vi "Test_Install_all_availablePXI.vi"(4 "error in":errorcluster, 7 "Parameter Array in":string[](array[string])) -> (0 "error out":errorcluster, 1 "Result Paragraphs":string[](array[string]), 2 "Pass":bool, 3 "Parameter Array Out":string[](array[string]))   [LabVIEW 2020]
uses:
  <vilib>/nisyscfg/Software 1.2.ctl
  <vilib>/nisyscfg/Component Type.ctl
  <vilib>/nisyscfg/Broken Dependency 1.2.ctl
  <vilib>/nisyscfg/Network Settings Format.ctl
  CommonSubVIs/Framework/Flattened_Array/Test Parameter Enum.ctl
  CommonSubVIs/Framework/Flattened_Array/Get Parameter Value by Name (String).vi
  <vilib>/nisyscfg/Get Filtered Base System Images.vi
  <vilib>/nisyscfg/Format With Base System Image.vi
  <vilib>/nisyscfg/Close (System).vi
  <vilib>/nisyscfg/nisyscfg.lvlib
  <resource>/objmgr/nisysapi.rc
panel:
  in  "Tab Control":enum32{"Connector Pane controls", "The rest"}(tab)
  in  "Network Address":string="10.0.62.162"
  out "Installed Software":T1[](array[typedef]) {"component type" items=["standard", "hidden", "system", "unknown", "startup", "image", "essential"]}
  out "Broken Dependencies":T3[](array[typedef]) {"dependee"."component type" items=["standard", "hidden", "system", "unknown", "startup", "image", "essential"]; "depender"."component type" items=["standard", "hidden", "system", "unknown", "startup", "image", "essential"]}
  in  "Network Settings (reset all adapters)":T4=1 items=["reset all network adapters", "preserve primary, reset others", "preserve all network adapters"]
  out "Base System Image":T1 caption="software" {"component type" items=["standard", "hidden", "system", "unknown", "startup", "image", "essential"]}
  # "This VI is used to install software to the Linux target USEING IPK"
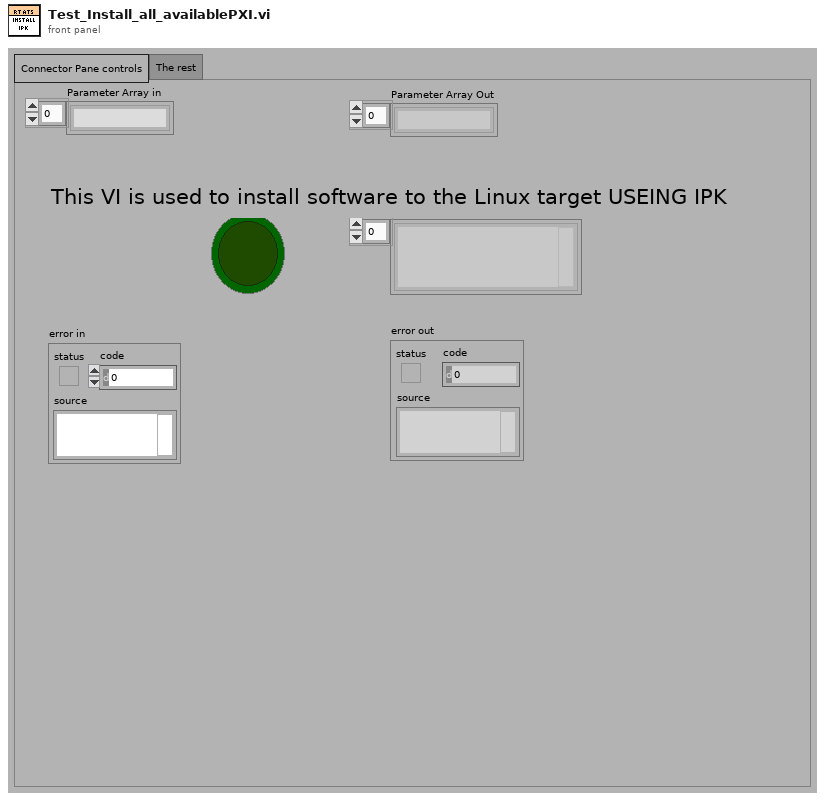
[diagram p1: front panel]
types:
  T1 = typedef "nisyscfg.lvlib/Software 1.2.ctl" = cluster{"title":string, "description":string, "ID":string, "version":string, "component type":T2}
  T2 = typedef "nisyscfg.lvlib/Component Type.ctl" = u32
  T3 = typedef "nisyscfg.lvlib/Broken Dependency 1.2.ctl" = cluster{"depender":T1, "dependee":T1}
  T4 = typedef "nisyscfg.lvlib/Network Settings Format.ctl" = u32
  T5 = typedef "Test Parameter Enum.ctl" = enum16{"Main Test Target IP", "Main Test Target Name", "Main Test Target Alias", "Main Host IP", "Default Target Alias", "Default Target Host Name", "Dafault Target IP Address", "Dafault Target LV Date", "Available Targets", "Target Alias by Index", "Target IP by Alias", "Target IP by  Index", "Current Iteration", "Total Iterations", "Test Project Name", "Current Test Result", "Current Test Name", "Current Test Logical Path", "Test Folder", "Configuration Name", "Configuration Index", "Total Configurations", "Performance Values", "Result Paragraphs", "Connector Pane", "Avoid?", "Avoid Reason", "Case Name", "Case #", "Total Cases", "Case Data", "Disable reason"}
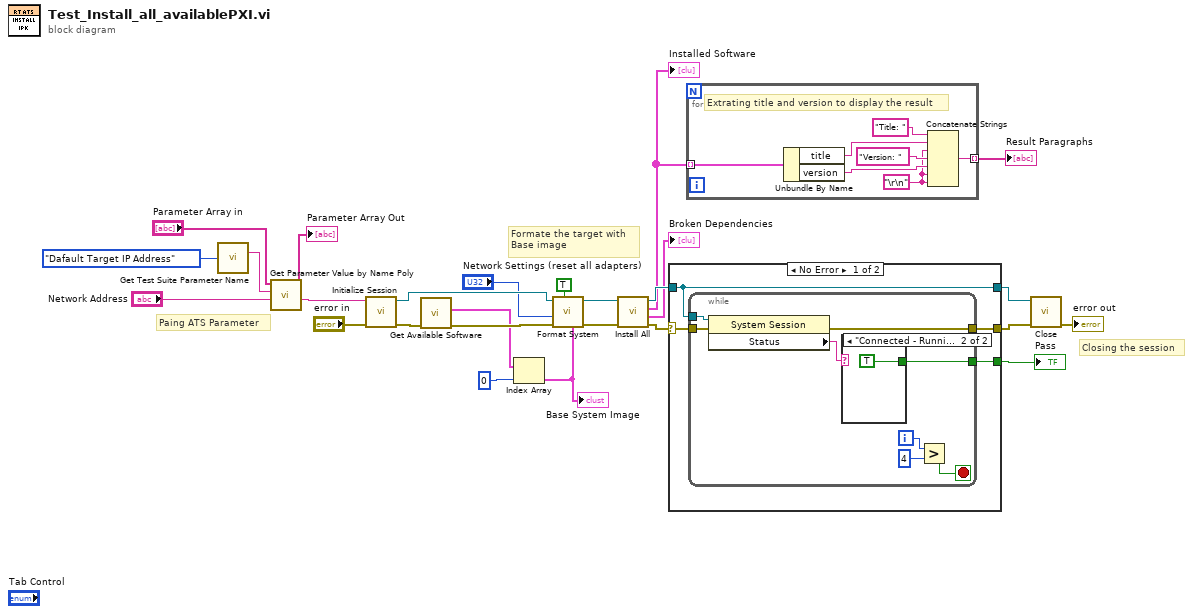
[diagram p0: block diagram]
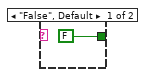
[diagram p2: hidden frame]
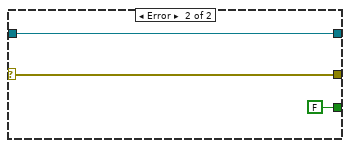
[diagram p3: hidden frame]
diagram:
  # "Closing the session"
  # "Paing ATS Parameter"
  # "Formate the target with \nBase image"
  n1 = call "Get Test Suite Parameter Name.vi"("Test Suite Parameter"=Test_Parameter_Enum."Dafault Target IP Address") -> ("Parameter Name"=w21:string)  [unwired: 13 in, 1 out]
  n2 = call-poly "Get Parameter Value by Name Poly.vi"("Default Value"="Network Address", "Parameter"=w21, "Parameter Array in"="Parameter Array in") -> ("Value"=w11:string, "Parameter Array Out"=→"Parameter Array Out":string[])  [unwired: 5 in, 1 out]
  n3 = call <vilib>:"Initialize Session.vi"("error in (no error)"="error in", "Target (localhost)"=w11) -> ("error out"=w5:errorcluster, "Session out"=w18:refnum<k21>)  [unwired: 8 in]
  n4 = call-poly <vilib>:"Get Available Software.vi"("error in (no error)"=w5) -> ("error out"=w4:errorcluster, "Base System Images"=w3:T1[])  [unwired: 8 in, 1 out]
  n5 = Index Array(array=w3, index=0) -> (element=w1:T1)
  "Base System Image" <- w1
  n6 = call-poly <vilib>:"Format System.vi"("Base System Image"=w1, "Restart Automatically (T)"=TRUE, "error in (no error)"=w4, "Network Settings (reset all adapters)"="Network Settings (reset all adapters)", "Session in"=w18) -> ("error out"=w16:errorcluster, "Session out"=w15:refnum<k21>)  [unwired: 5 in]
  n7 = call <vilib>:"Install All.vi"("error in (no error)"=w16, "Session in"=w15) -> ("error out"=w24:errorcluster, "Broken Dependencies"=→"Broken Dependencies":T3[], "Installed Software"=w7:T1[], "Session out"=w25:refnum<k21>)  [unwired: 6 in]
  "Installed Software" <- w7
  n8 = case shown="No Error" w24 {
    selector: w24 -> [w29 w41]
    tunnel: w25 -> [w27 w43]
    tunnel: [w30 FALSE] -> w26
    tunnel: [w27 w43] -> w12
    tunnel: [w28 w41] -> w14
    frame No Error {
      n9 = while {
        tunnel: w29 -> [w34]
        tunnel: [w31] -> w28
        tunnel: [w38] -> w30
        tunnel: w27 -> [w33]
        i -> [w37]
        stop <- w35 stop-if-true
        n10 = property class="System Session"(reference=w33, error in=w34) -> (error out=w31:errorcluster, "Status"=w32:string)  [unwired: 1 out]
        n11 = case shown="\"Connected - Running\"" w32 {
          tunnel: [FALSE TRUE] -> w38
          frame "False", Default {
          }
          frame "Connected - Running" {
          }
        }
        n12 = Greater?(x=w37, y=4) -> (0:w35:bool)
      }
    }
    frame Error {
    }
  }
  "Pass" <- w26
  n13 = for {
    tunnel: w7 -> [w50] mode=indexing
    tunnel: [w45] -> w6 mode=indexing
    w44 = "\r\n"
    # "Extrating title and version to display the result"
    n14 = Unbundle By Name(w50) -> ("title"=w48:string, "version"=w46:string)
    n15 = Concatenate Strings("Title: " ("string"), w48, w44, "Version: " ("string"), w46, w44, w44) -> (w45:string)
  }
  "Result Paragraphs" <- w6
  n16 = call-poly <vilib>:"Close.vi"("error in (no error)"=w14, "Session in"=w12) -> ("error out"=→"error out":errorcluster)  [unwired: 9 in]
